vi "rs3_close all.vi"(6 "rscontext":u64, 7 "queue in":u64, 8 "error in (no error)":errorcluster, 9 "device_list":u64, 10 "Dev in":u64, 11 "Sensor in":u64) -> (0 "error out (no error)":errorcluster, 3 "Close Error":string)   [LabVIEW 2023]
doc: "It is important to close everything properly at the end. Use this VI to clean up and close the RealSense device, queue, sensor, and device list."
panel:
  # "RS3 Close All"
  # "(C) Intel Corp. 2017,  AGJ"
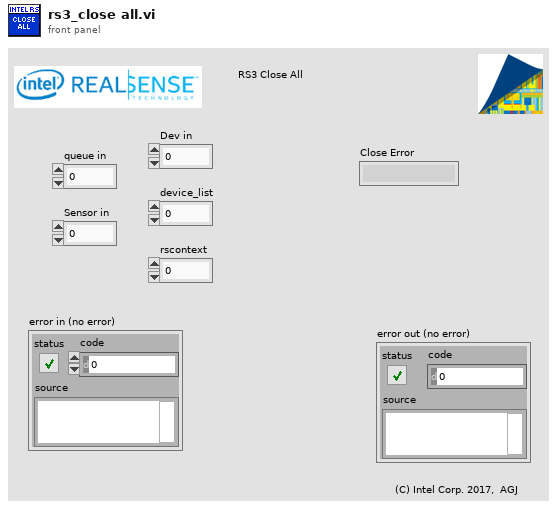
[diagram p1: front panel]
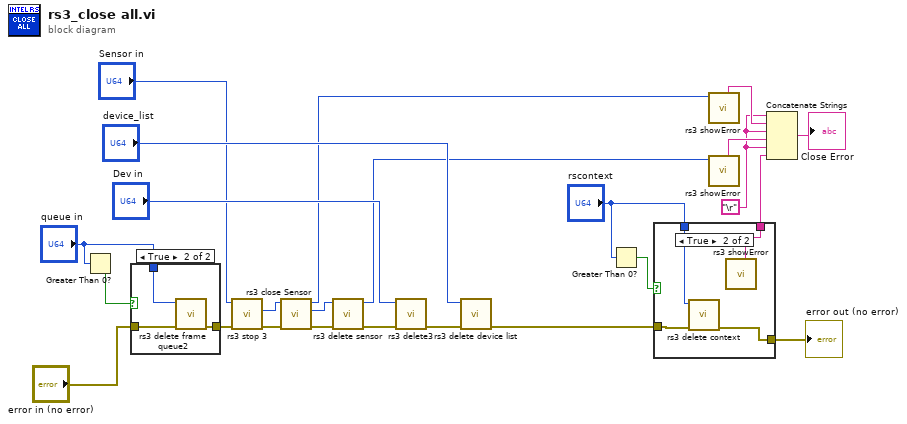
[diagram p0: block diagram]
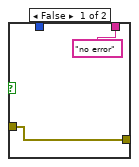
[diagram p3: hidden frame]
diagram:
  w5 = "\r"
  n1 = Greater Than 0?(x="queue in") -> (x > 0?=w3:bool)
  n2 = case shown="True" w3 {
    tunnel: "error in (no error)" -> [w25 w28]
    tunnel: "queue in" -> [_ w27]
    tunnel: [w25 w26] -> w9
    frame False {
    }
    frame True {
      n3 = call "rs3 delete frame queue2.vi"("error in (no error)"=w28, "queue"=w27) -> ("error out"=w26:errorcluster)  [unwired: 9 in]
    }
  }
  n4 = call "rs3 stop 3.vi"("error in (no error)"=w9, "device"="Sensor in") -> ("error out"=w8:errorcluster, "device out"=w6:u64)  [unwired: 8 in]
  n5 = call "rs3 close Sensor.vi"("error in (no error)"=w8, "sensor"=w6) -> ("error out"=w22:errorcluster, "device out"=w21:u64, "error"=w12:u64)  [unwired: 7 in]
  n6 = call "rs3 delete sensor.vi"("error in (no error)"=w22, "sensor"=w21) -> ("error out"=w23:errorcluster, "error"=w11:u64)  [unwired: 8 in]
  n7 = call "rs3 delete3.vi"("error in (no error)"=w23, "device"="Dev in") -> ("error out"=w18:errorcluster)  [unwired: 9 in]
  n8 = call "rs3 delete device list.vi"("error in (no error)"=w18, "device list"="device_list") -> ("error out"=w20:errorcluster)  [unwired: 9 in]
  n9 = Greater Than 0?(x="rscontext") -> (x > 0?=w1:bool)
  n10 = case shown="True" w1 {
    tunnel: w20 -> [w29 w34]
    tunnel: [w29 w33] -> w16
    tunnel: ["no error" ("Error summary") w32] -> w10
    tunnel: "rscontext" -> [_ w31]
    frame False {
    }
    frame True {
      n11 = call "rs3 delete context.vi"("error in (no error)"=w34, "context"=w31) -> ("error out"=w33:errorcluster)  [unwired: 9 in]
      n12 = call "rs3 showError.vi"() -> ("Error summary"=w32:string)  [unwired: 7 in, 4 out]
    }
  }
  "error out (no error)" <- w16
  n13 = call "rs3 showError.vi"("error"=w12) -> ("Error summary"=w15:string)  [unwired: 6 in, 4 out]
  n14 = call "rs3 showError.vi"("error"=w11) -> ("Error summary"=w14:string)  [unwired: 6 in, 4 out]
  n15 = Concatenate Strings(w5, w15, w5, w14, w5, w10) -> (→"Close Error":string)
